vi "Read Power.vi"(8 "error in (no error)":errorcluster, 11 "Power Meter in":refnum<class "Power Meter.lvclass">) -> (0 "error out":errorcluster, 1 "Current Power w/ Units":string, 2 "Current Power":dbl[unit], 3 "Power Meter out":refnum<class "Power Meter.lvclass">)   [LabVIEW 2009, in "Power Meter.lvclass"]
doc: "Public Interface for _Read.vi\nReturns the Power as SI formatted string with \"W\" appended."
uses:
  Power Meter.lvclass
  Power Meter.lvclass/Power Meter.ctl
  Newport 1830-C/Newport 1830-C.lvlib
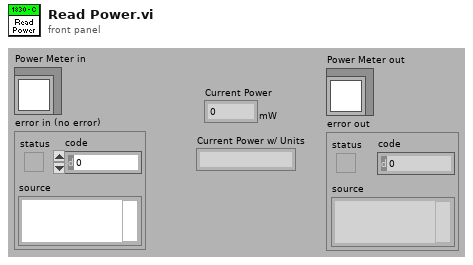
[diagram p1: front panel]
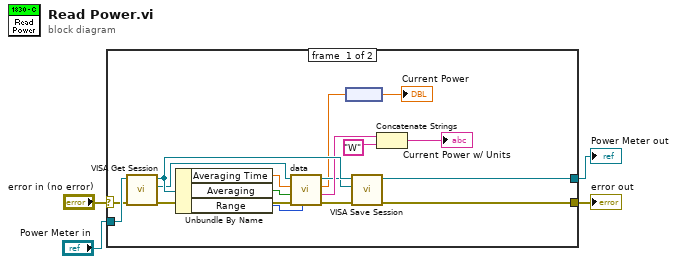
[diagram p0: block diagram]
diagram:
  n1 = case shown="No Error" "error in (no error)" {
    selector: "error in (no error)" -> [w20 w22]
    tunnel: "Power Meter in" -> [w21 w23]
    tunnel: [w19 w22] -> w2
    tunnel: [w18 w23] -> w1
    frame #0 {
      n2 = call-dynamic "VISA Get Session.vi"("error in (no error)"=w20, "Instrument.lvclass in"=w21) -> ("error out"=w14:errorcluster, "VISA Resource Name"=w15:refnum<visa-resource-name>, "Instrument.lvclass out"=w17:refnum<class "Power Meter.lvclass">)  [unwired: 7 out]
      n3 = Unbundle By Name(w17) -> ("Averaging Time"=w13:dbl, "Averaging"=w12:bool, "Range"=w5:u16)
      n4 = call "data.vi"("Current Range"=w5, "error in (no error)"=w14, "AVG?"=w12, "Averaging Time"=w13, "VISA resource name"=w15) -> ("error out"=w8:errorcluster, "SI"=w11:string, "output"=w6:dbl, "VISA resource name out"=w9:refnum<visa-resource-name>)  [unwired: 3 in]
      n5 = node(w6) -> (→"Current Power":dbl[unit])
      n6 = call-dynamic "VISA Save Session.vi"("error in (no error)"=w8, "VISA Resource Name"=w9, "Instrument.lvclass in"=w17) -> ("error out"=w19:errorcluster, "Instrument.lvclass out"=w18:refnum<class "Power Meter.lvclass">)  [unwired: 7 out]
      n7 = Concatenate Strings(w11, "W" ("string")) -> (→"Current Power w/ Units":string)
    }
    frame #1 {
    }
  }
  "error out" <- w2
  "Power Meter out" <- w1
